vi "Start_LDA.vi"() -> ()   [LabVIEW 2012]
doc: "The Getting Started Analog Input VI illustrates the basic concepts involved in acquiring analog input data from any data acquisition hardware.\n\nThis VI is explained in detail in the Getting Started with Analog Input section of chapter 1 of the Data Acquisition VI Reference Manual. If you are using SCXI, you should read the Getting Started with SCXI section of chapter 1 first.\n\nAfter you have installed and configured your data acquisition hardware as described in the Installation and Configuration section of chapter 1, you can run this VI to verify your hardware configuration. \n\nYou can pop-up on any front panel object for a description.\n\nIf you are using AMUX-64T boards or SCXI hardware, look at the channels control description for instructions on how to address those external channels; otherwise, you can run the VI with default inputs.\n\nOpen the diagram window to see the data acquisition VI usage."
uses:
  Globals/LDA_meas_global_1.vi
  Globals/Meas_global.vi
  Globals/LDA_meas_global_2.vi
panel:
  in  "Hold for PW to fire (ms)":u32
  out "error out":errorcluster
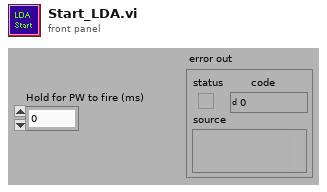
[diagram p1: front panel]
types:
  T1 = typedef "BSA_info_Cluster.ctl" = cluster{"GPIB Address":string, "No of Check Bytes":i32, "Extra Info":string, "COLOUR":u32, "Wavelength (nm)":dbl}
  T2 = typedef "LDA_Setup.ctl" = cluster{"dimensions":enum16{"1D", "2D"}, "Analogue Freq Multiplier":dbl}
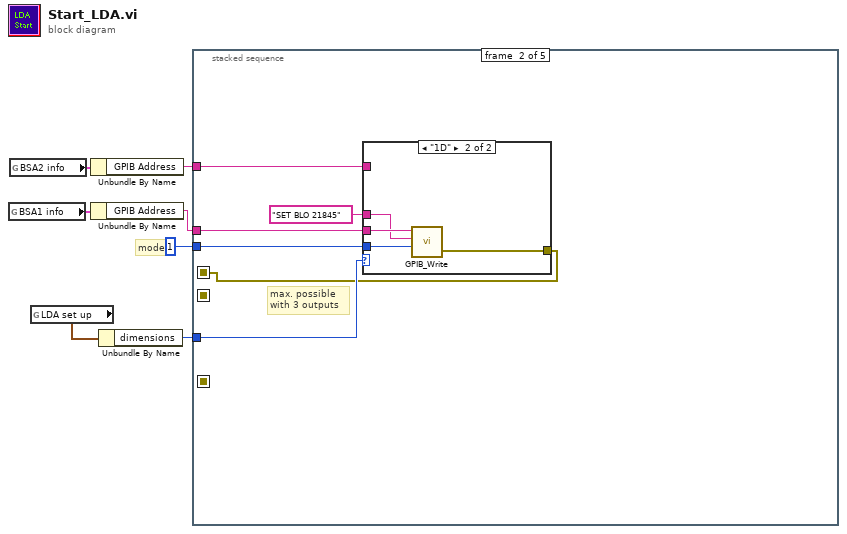
[diagram p0: block diagram]
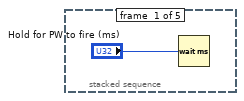
[diagram p2: hidden frame]
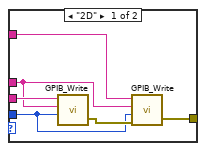
[diagram p3: hidden frame]
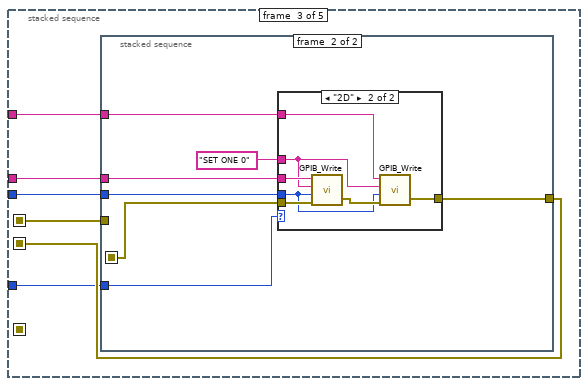
[diagram p4: hidden frame]
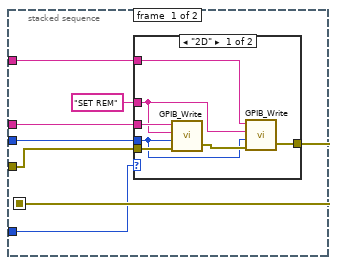
[diagram p5: hidden frame]
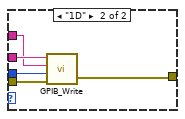
[diagram p6: hidden frame]
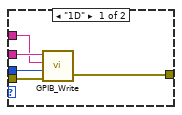
[diagram p7: hidden frame]
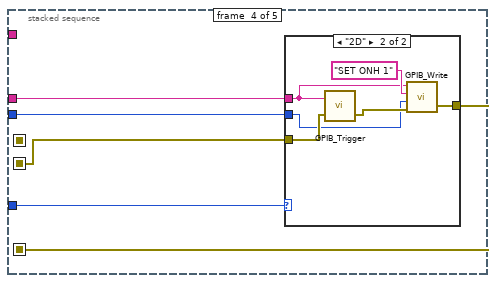
[diagram p8: hidden frame]
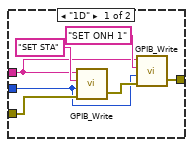
[diagram p9: hidden frame]
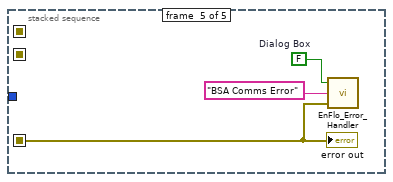
[diagram p10: hidden frame]
diagram:
  # "mode"
  n1 = global read "LDA_meas_global_1.vi" "BSA1 info"() -> (w4:T1)
  n2 = global read "LDA_meas_global_2.vi" "BSA2 info"() -> (w3:T1)
  n3 = global read "Meas_global.vi" "LDA set up"() -> (w2:T2)
  n4 = Unbundle By Name(w3) -> ("GPIB Address"=w5:string)
  n5 = Unbundle By Name(w4) -> ("GPIB Address"=w6:string)
  n6 = Unbundle By Name(w2) -> ("dimensions"=w1:enum16{"1D", "2D"})
  n7 = stacked-sequence {
    seq-local: [_ w9 _ _ _] -> [_ _ w28 _ _]
    seq-local: [_ _ w27 _ _] -> [_ _ _ w71 _]
    seq-local: [_ _ _ w70 _] -> [_ _ _ _ w87]
    tunnel: w6 -> [_ w14 w29 w69 _]
    tunnel: i16 1 -> [_ w12 w30 w72 _]
    tunnel: w1 -> [_ w11 w26 w73 _]
    tunnel: w5 -> [_ w10 w25 _ _]
    frame #0 {
      n8 = Wait (ms)(milliseconds to wait="Hold for PW to fire (ms)") -> ()  [unwired: 1 out]
    }
    frame #1 {
      # "max. possible with 3 outputs"
      n9 = case shown="\"1D\"" w11 {
        tunnel: w14 -> [w20 w24]
        tunnel: "SET BLO 21845" -> [w18 w22]
        tunnel: w12 -> [w17 w23]
        tunnel: w10 -> [w16 _]
        tunnel: [w15 w21] -> w9
        frame "2D" {
          n10 = call "GPIB_Write.vi"("address string"=w20, "data In"=w18, "mode (0)"=w17) -> ("error out"=w19:errorcluster)  [unwired: 2 in, 1 out]
          n11 = call "GPIB_Write.vi"("address string"=w16, "data In"=w18, "mode (0)"=w17, "error in"=w19) -> ("error out"=w15:errorcluster)  [unwired: 1 in, 1 out]
        }
        frame "1D" {
          n12 = call "GPIB_Write.vi"("address string"=w24, "data In"=w22, "mode (0)"=w23) -> ("error out"=w21:errorcluster)  [unwired: 2 in, 1 out]
        }
      }
    }
    frame #2 {
      n13 = stacked-sequence {
        seq-local: [w32 _] -> [_ w54]
        tunnel: w30 -> [w36 w56]
        tunnel: w29 -> [w37 w55]
        tunnel: w28 -> [w35 _]
        tunnel: [_ w53] -> w27
        tunnel: w26 -> [w31 w52]
        tunnel: w25 -> [w33 w50]
        frame #0 {
          n14 = case shown="\"2D\"" w31 {
            tunnel: w37 -> [w44 w49]
            tunnel: w36 -> [w41 w47]
            tunnel: w35 -> [w43 w48]
            tunnel: "SET REM" -> [w40 w46]
            tunnel: w33 -> [w39 _]
            tunnel: [w38 w45] -> w32
            frame "2D" {
              n15 = call "GPIB_Write.vi"("address string"=w44, "data In"=w40, "mode (0)"=w41, "error in"=w43) -> ("error out"=w42:errorcluster)  [unwired: 1 in, 1 out]
              n16 = call "GPIB_Write.vi"("address string"=w39, "data In"=w40, "mode (0)"=w41, "error in"=w42) -> ("error out"=w38:errorcluster)  [unwired: 1 in, 1 out]
            }
            frame "1D" {
              n17 = call "GPIB_Write.vi"("address string"=w49, "data In"=w46, "mode (0)"=w47, "error in"=w48) -> ("error out"=w45:errorcluster)  [unwired: 1 in, 1 out]
            }
          }
        }
        frame #1 {
          n18 = case shown="\"2D\"" w52 {
            tunnel: w56 -> [w61 w65]
            tunnel: w55 -> [w60 w68]
            tunnel: w54 -> [w59 w67]
            tunnel: [w58 w62] -> w53
            tunnel: "SET ONE 0" -> [w57 w63]
            tunnel: w50 -> [_ w64]
            frame "1D" {
              n19 = call "GPIB_Write.vi"("address string"=w60, "data In"=w57, "mode (0)"=w61, "error in"=w59) -> ("error out"=w58:errorcluster)  [unwired: 1 in, 1 out]
            }
            frame "2D" {
              n20 = call "GPIB_Write.vi"("address string"=w68, "data In"=w63, "mode (0)"=w65, "error in"=w67) -> ("error out"=w66:errorcluster)  [unwired: 1 in, 1 out]
              n21 = call "GPIB_Write.vi"("address string"=w64, "data In"=w63, "mode (0)"=w65, "error in"=w66) -> ("error out"=w62:errorcluster)  [unwired: 1 in, 1 out]
            }
          }
        }
      }
    }
    frame #3 {
      n22 = case shown="\"2D\"" w73 {
        tunnel: w69 -> [w74 w81]
        tunnel: w72 -> [w75 w82]
        tunnel: w71 -> [w80 w84]
        tunnel: [w76 w85] -> w70
        frame "1D" {
          n23 = call "GPIB_Write.vi"("address string"=w74, "data In"="SET STA", "mode (0)"=w75, "error in"=w80) -> ("error out"=w77:errorcluster)  [unwired: 1 in, 1 out]
          n24 = call "GPIB_Write.vi"("address string"=w74, "data In"="SET ONH 1", "mode (0)"=w75, "error in"=w77) -> ("error out"=w76:errorcluster)  [unwired: 1 in, 1 out]
        }
        frame "2D" {
          n25 = call "GPIB_Trigger.vi"("error in"=w84, "address string"=w81) -> ("error out"=w83:errorcluster)  [unwired: 1 out]
          n26 = call "GPIB_Write.vi"("address string"=w81, "data In"="SET ONH 1", "mode (0)"=w82, "error in"=w83) -> ("error out"=w85:errorcluster)  [unwired: 1 in, 1 out]
        }
      }
    }
    frame #4 {
      w89 = FALSE  # Dialog Box
      n27 = call "EnFlo_Error_Handler.vi"("error in (no error)"=w87, "Error Type"="BSA Comms Error", "Dialog Box (T)"=w89) -> ()  [unwired: 3 out]
      "error out" <- w87
    }
  }
